vi "Drive Controller.vi"(8 "error in":errorcluster) -> ()   [LabVIEW 2016]
doc: "This VI executes continuously carrying out the current operation and responding to updates or new operation requests. It will often contain the timing or control code that is difficult to place directly in TeleOp. This VI generally opens all sensors and motors and isolates the rest of the robot code from knowing implementation details of how the operations are carried out."
uses:
  Drive Setpoints.ctl
  Drive Operations.ctl
  <vilib>/Rock Robotics/WPI/SafetyOutput/WPI_SafetyOutputConfigMenu.ctl
  <vilib>/Rock Robotics/WPI/Utilities/WPI_GetSetVariantRefNum.vi
panel:
  out "Setpoints":T1(graph)
  out "Current\nCmd":string
  # "Tip: It may be helpful to observe inputs and sensor values.\nYou may also want to display tuning or debugging controls."
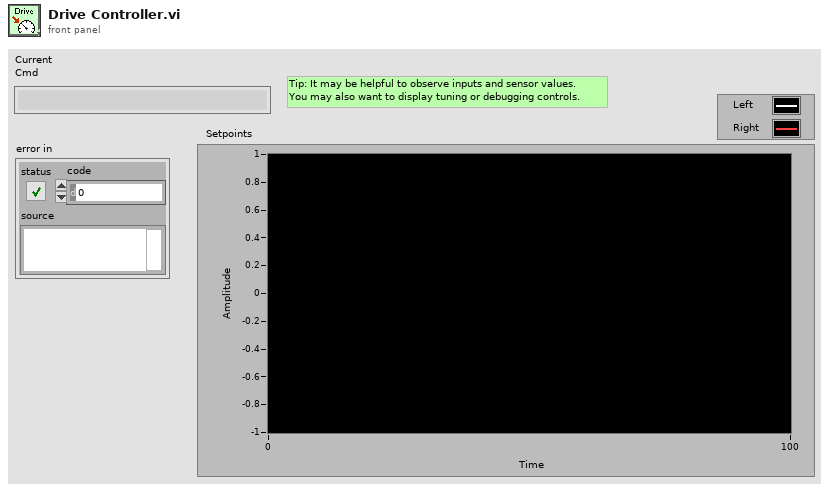
[diagram p1: front panel]
types:
  T1 = cluster{"Left Setpoint":dbl, "Right Setpoint":dbl}
  T2 = typedef "WPI_SafetyOutputConfigMenu.ctl" = enum16{"Enable", "Disable"}
  T3 = typedef "Drive Setpoints.ctl" = cluster{"Operation":T4, "Left Setpoint":dbl, "Right Setpoint":dbl, "Duration":dbl}
  T4 = typedef "Drive Operations.ctl" = enum16{"Reserve", "Read Current", "Immediate", "Drive for Time", "Drive for Distance"}
  T5 = typedef "WPI_RobotDriveDevRef.ctl" = cluster{"DevStatus":errorcluster, "Motors[]":T6[], "Square Inputs":bool, "Max Output":dbl}
  T6 = typedef "WPI_MotorControlDeviceRef.ctl" = cluster{"DeviceStatus":errorcluster, "Type":T7, "PWM":cluster{"PWM Channel":T8, "DeadBand":T9}, "CAN":cluster{"Device Number":u8, "SetOutput VI Ref":variant, "GetOutput VI Ref":variant, "Enable VI Ref":variant, "Disable VI Ref":variant, "Data":variant}, "Invert":bool}
  T7 = typedef "WPI_MotorControlType.ctl" = enum16{"PWM", "CAN"}
  T8 = typedef "FPGA_DIOPWMChannel.ctl" = enum8{"PWM 0", "PWM 1", "PWM 2", "PWM 3", "PWM 4", "PWM 5", "PWM 6", "PWM 7", "PWM 8", "PWM 9", "PWM MXP 0", "PWM MXP 1", "PWM MXP 2", "PWM MXP 3", "PWM MXP 4", "PWM MXP 5", "PWM MXP 6", "PWM MXP 7", "PWM MXP 8", "PWM MXP 9", "Invalid"}
  T9 = typedef "WPI_PWMDeadband.ctl" = cluster{"Name":string, "maxPositivePwm":i32, "minPositivePwm":i32, "centerPwm":i32, "maxNegativePwm":i32, "minNegativePwm":i32, "angularRange":u16}
  T10 = typedef "Command Status Info.ctl" = cluster{"Name":string, "Status":T11, "notifier out":T12}
  T11 = typedef "Completion Status.ctl" = enum16{"Successful", "Aborted", "Incomplete"}
  T12 = typedef "Completion Notifier.ctl" = refnum<notifier>
  T13 = cluster{"SubSystem Data":T3, cluster{"Start Time (ms)":u32, "Iterations":i32}, cluster{"Command Info":T10, "Description":string, "SubSystem Data":T3, "notifier out":refnum<notifier>, "Subsystem Name":string}}
  T14 = cluster{"SubSystem Data":T3, cluster{"Start Time (ms)":u32, "Iterations":i32}, "Default Command Arguments":cluster{"Command Info":T10, "Description":string, "SubSystem Data":T3, "notifier out":refnum<notifier>, "Subsystem Name":string}}
  T15 = cluster{"Don't move motors while reserved":dbl, "Don't move motors while reserved":dbl}
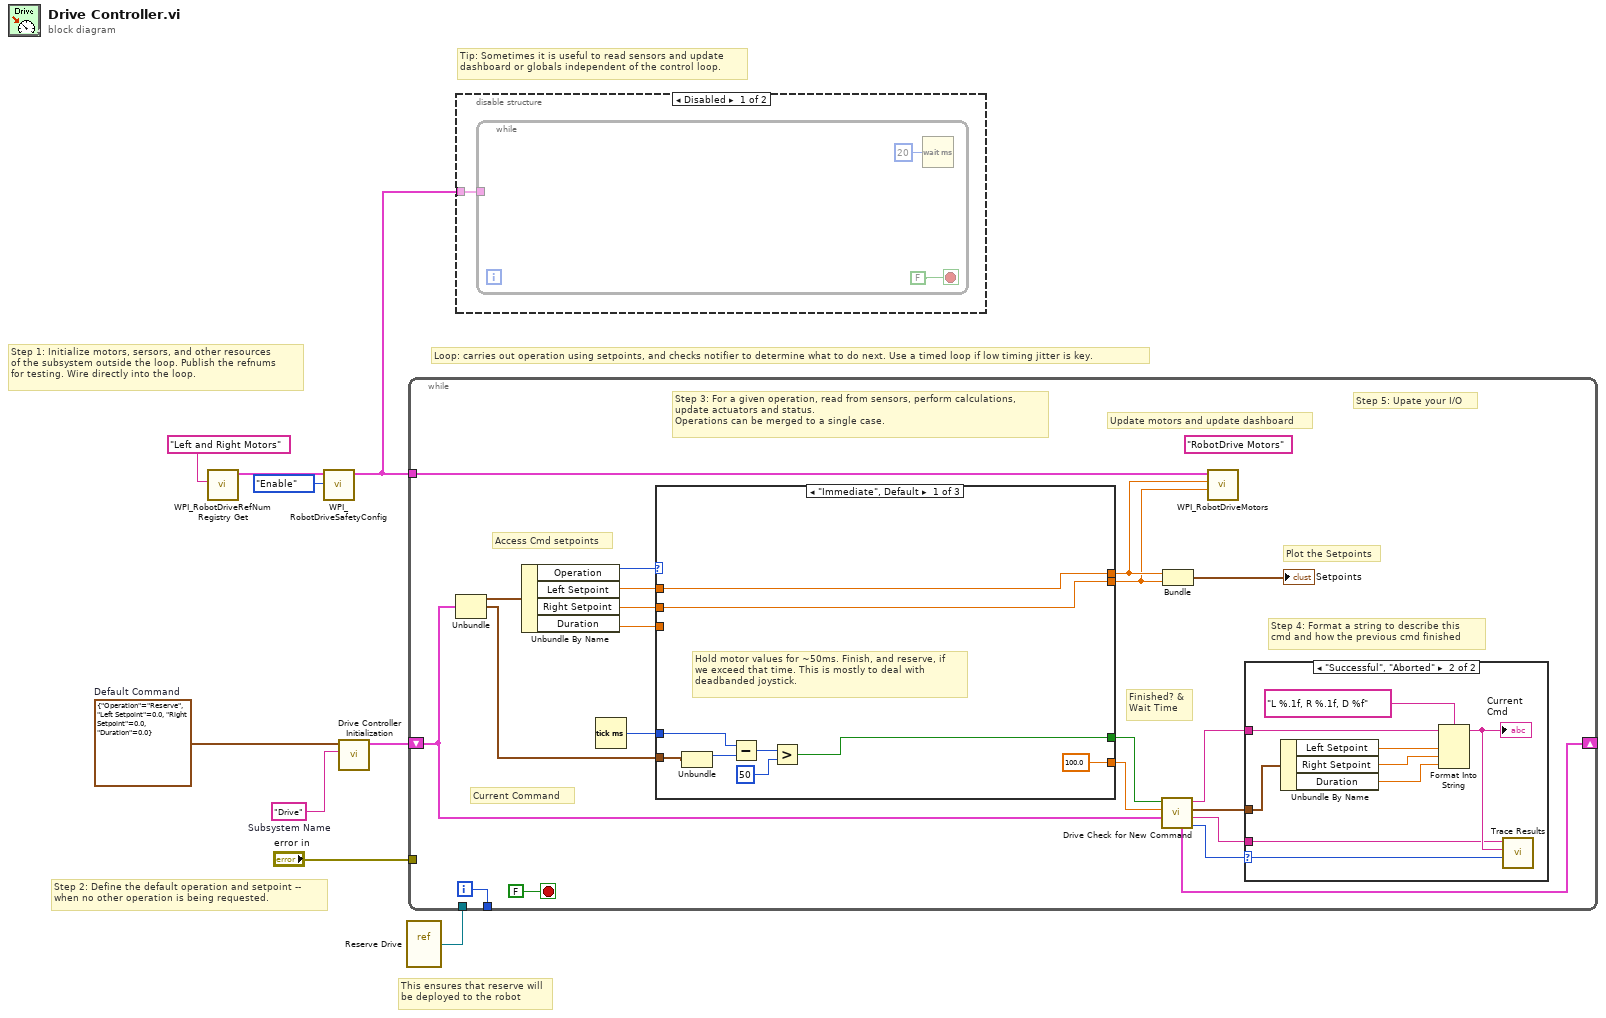
[diagram p0: block diagram]
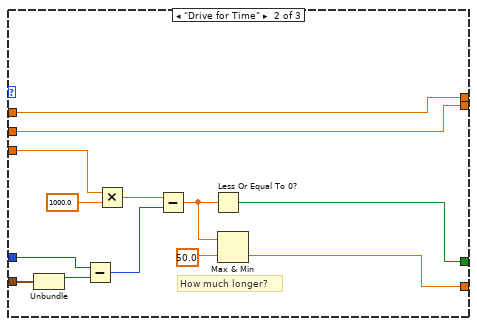
[diagram p4: hidden frame]
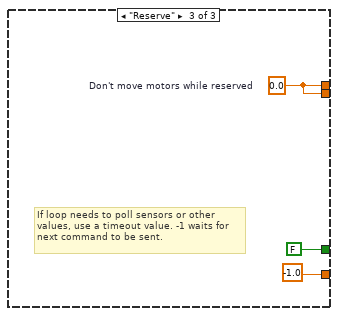
[diagram p5: hidden frame]
diagram:
  w8 = T3 {"Operation"=enum."Reserve", "Left Setpoint"=0.0, "Right Setpoint"=0.0, "Duration"=0.0}  # Default Command
  w9 = "Drive"  # Subsystem Name
  # "This ensures that reserve will\nbe deployed to the robot"
  # "Tip: Sometimes it is useful to read sensors and update\ndashboard or globals independent of the control loop."
  # "Step 2: Define the default operation and setpoint --\nwhen no other operation is being requested."
  # "Step 1: Initialize motors, sersors, and other resources\nof the subsystem outside the loop. Publish the refnums\nfor testing. Wire directly into the loop."
  # "Loop: carries out operation using setpoints, and checks notifier to determine what to do next. Use a timed loop if low timing jitter is key."
  n1 = call <vilib>:"WPI_RobotDriveRefNum Registry Get.vi"("refnum name"="Left and Right Motors") -> ("RobotDriveDevRef"=w6:T5)  [unwired: 9 in, 1 out]
  n2 = call <vilib>:"WPI_RobotDriveSafetyConfig.vi"("mode"=WPI_SafetyOutputConfigMenu."Enable", "RobotDriveDevRef"=w6) -> ("RobotDriveDevRef"=w4:T5)  [unwired: 8 in, 1 out]
  n3 = call "Drive Controller Initialization.vi"("Subsystem Name"=w9, "Default Command"=w8) -> ("output cluster"=w2:T13)  [unwired: 9 in]
  n4 = vi-ref "Reserve Drive.vi"() -> (w1:refnum<vi>)
  n5 = while {
    shift-right: [w17] -> _
    shift-left: w2 -> [w10]
    tunnel: [w29] -> _
    tunnel: w4 -> [w25]
    tunnel: "error in" -> [_]
    tunnel: w1 -> [_]
    i -> [w29]
    stop <- FALSE stop-if-true
    (unwired) "RobotDrive Motors" ("Name")
    # "Step 5: Upate your I/O"
    # "Step 4: Format a string to describe this\ncmd and how the previous cmd finished"
    # "Current Command"
    # "Update motors and update dashboard"
    # "Plot the Setpoints"
    # "Access Cmd setpoints"
    # "Finished? &\nWait Time"
    # "Step 3: For a given operation, read from sensors, perform calculations,\nupdate actuators and status.\nOperations can be merged to a single case."
    n6 = Unbundle(w10) -> ("SubSystem Data"=w24:T3, w11:cluster{"Start Time (ms)":u32, "Iterations":i32})  [unwired: 1 out]
    n7 = Unbundle By Name(w24) -> ("Operation"=w23:T4, "Left Setpoint"=w22:dbl, "Right Setpoint"=w21:dbl, "Duration"=w20:dbl)
    n8 = Tick Count (ms)() -> (millisecond timer value=w19:u32)
    n9 = case shown="\"Immediate\", Default" w23 {
      tunnel: [100.0 w49 -1.0] -> w16
      tunnel: [w41 w56 FALSE ("ignore previous (F)")] -> w15
      tunnel: w11 -> [w40 w58 _]
      tunnel: [w47 w55 w62] -> w27
      tunnel: [w46 w54 w62] -> w26
      tunnel: w22 -> [w47 w55 _]
      tunnel: w21 -> [w46 w54 _]
      tunnel: w20 -> [_ w53 _]
      tunnel: w19 -> [w42 w52 _]
      frame "Immediate", Default {
        # "Hold motor values for ~50ms. Finish, and reserve, if\nwe exceed that time. This is mostly to deal with\ndeadbanded joystick."
        n10 = Unbundle(w40) -> ("Start Time (ms)"=w43:u32)  [unwired: 1 out]
        n11 = Subtract(x=w42, y=w43) -> (x-y=w44:u32)
        n12 = Greater?(x=w44, y=u8 50 ("Left Motor")) -> (0:w41:bool)
      }
      frame "Drive for Time" {
        # "How much longer?"
        n13 = Unbundle(w58) -> ("Start Time (ms)"=w57:u32)  [unwired: 1 out]
        n14 = Subtract(x=w52, y=w57) -> (x-y=w61:u32)
        n15 = Multiply(x=w53, y=1000.0) -> (x*y=w60:dbl)
        n16 = Subtract(x=w60, y=w61) -> (x-y=w51:dbl)
        n17 = Less Or Equal To 0?(x=w51) -> (x <= 0?=w56:bool)
        n18 = Max & Min(x=w51, y=50.0) -> (min(x,y)=w49:dbl)  [unwired: 1 out]
      }
      frame "Reserve" {
        w62 = 0.0  # Don't move motors while reserved
        # "If loop needs to poll sensors or other\nvalues, use a timeout value. -1 waits for\nnext command to be sent."
      }
    }
    n19 = call "Drive Check for New Command.vi"("input cluster"=w10, "Wait time (ms)"=w16, "Finished?"=w15) -> ("Completion"=w18:T11, "Subsystem Name"=w12:string, "SetPoint"=w13:T3, "Initial Trace String"=w14:string, "output cluster"=w17:T14)  [unwired: 4 in]
    n20 = Bundle("Don't move motors while reserved"=w27, "Don't move motors while reserved"=w26) -> (→"Setpoints":T15)  [unwired: 1 in]
    n21 = call <vilib>:"WPI_RobotDriveMotors.vi"("RightSpeed"=w26, "LeftSpeed"=w27, "RobotDriveDevRef"=w25) -> ()  [unwired: 1 in, 8 out]
    n22 = case shown="\"Successful\", \"Aborted\"" w18 {
      selector: w18 -> [_ w39]
      tunnel: w14 -> [_ w34]
      tunnel: w13 -> [_ w35]
      tunnel: w12 -> [_ w31]
      frame "Incomplete", Default {
        # "Continuing current command"
      }
      frame "Successful", "Aborted" {
        # "Report and setup for next command"
        n23 = Unbundle By Name(w35) -> ("Left Setpoint"=w37:dbl, "Right Setpoint"=w38:dbl, "Duration"=w32:dbl)
        n24 = Format Into String(format string="L %.1f, R %.1f, D %f", initial string=w34, w37, w38, w32) -> (resulting string=w33:string)  [unwired: 1 in, 1 out]
        "Current\nCmd" <- w33
        n25 = call <vilib>:"Trace Results.vi"("Status of previous command"=w39, "Description"=w33, "Subsystem"=w31) -> ()  [unwired: 9 in]
      }
    }
  }
  n26 = disable-structure shown="Disabled" {
    disable-tunnel: w4 -> [w65 _]
    frame Disabled {
      n27 = while {
        tunnel: w65 -> [_]
        stop <- FALSE stop-if-true
        n28 = Wait (ms)(milliseconds to wait=u32 20) -> ()  [unwired: 1 out]
      }
    }
    frame Enabled {
    }
  }
